vi "RQST Comm_Close All Connections.vi"(7 "Name":string, 8 "error in":errorcluster, 10 "ref in":T1, 11 "listener ID":refnum<k5>) -> (0 "error out":errorcluster)   [LabVIEW 2015, in "Diagnostics Addon Engine.lvlib"]
uses:
  Diagnostics Addon Engine.lvlib
  STM Lookup Table Ref.ctl
  Connection Manager/stm_TCPConnectionMethod.ctl
  <vilib>/NI Veristand/Custom Device Tools/Custom Device Utility Library/Custom Device Utility Library.lvlib
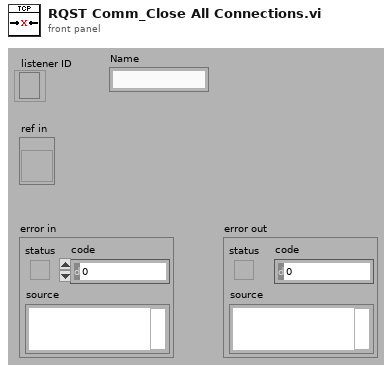
[diagram p1: front panel]
types:
  T1 = typedef "Diagnostics Addon Engine.lvlib/STM Lookup Table Ref.ctl" = refnum<vi>
  T2 = typedef "Diagnostics Addon Engine.lvlib/stm_TCPConnectionMethod.ctl" = enum16{"Initialize", "Add Connection", "Set Properties", "Get Connection(s)", "Remove Connection", "Remove All Connections", "Get Connection Count"}
  T3 = typedef "Diagnostics Addon Engine.lvlib/stm_TCP Connection Info.ctl" = cluster{"connection ID":refnum<k5>, "Meta data":T4[]}
  T4 = typedef "Diagnostics Addon Engine.lvlib/stm_MetaDataElement.ctl" = string
  T5 = typedef "Diagnostics Addon Engine.lvlib/stm_TCPConnectionProperties.ctl" = cluster{"Name":string, "Address":string, "Custom":string}
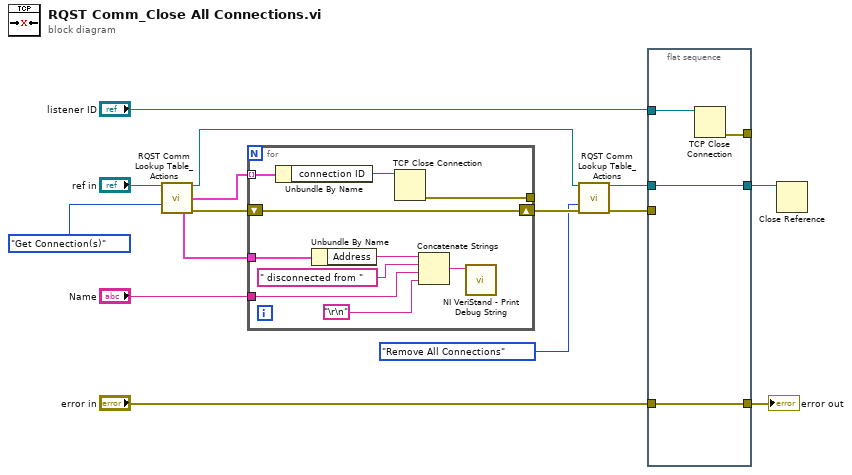
[diagram p0: block diagram]
diagram:
  n1 = call "RQST Comm Lookup Table_Actions.vi"("ref in"="ref in", "Method"=stm_TCPConnectionMethod."Get Connection(s)") -> ("ref out"=w3:T1, "All Connections"=w11:T3[], "Properties Out"=w1:T5, "error out"=w10:errorcluster)  [unwired: 7 in, 3 out]
  n2 = for {
    tunnel: w11 -> [w17] mode=indexing
    shift-right: [w23] -> w9
    shift-left: w10 -> [w23]
    tunnel: [w24] -> _
    tunnel: "Name" -> [w19]
    tunnel: w1 -> [w18]
    n3 = Unbundle By Name(w17) -> ("connection ID"=w25:refnum<k5>)
    n4 = Unbundle By Name(w18) -> ("Address"=w20:string)
    n5 = TCP Close Connection(connection ID=w25) -> (error out=w24:errorcluster)  [unwired: 2 in, 1 out]
    n6 = Concatenate Strings(w20, " disconnected from " ("string"), w19, "\r\n") -> (w22:string)
    n7 = call <vilib>:"NI VeriStand - Print Debug String.vi"("Message"=w22) -> ()  [unwired: 10 in, 1 out]
  }
  n8 = call "RQST Comm Lookup Table_Actions.vi"("ref in"=w3, "Method"=stm_TCPConnectionMethod."Remove All Connections", "error in (no error)"=w9) -> ("ref out"=w5:T1, "error out"=w8:errorcluster)  [unwired: 6 in, 5 out]
  n9 = flat-sequence {
    tunnel: "listener ID" -> [w29]
    tunnel: [w28] -> w14
    tunnel: w8 -> [_]
    tunnel: "error in" -> [w28]
    tunnel: [w27] -> _
    tunnel: w5 -> [w26]
    tunnel: [w26] -> w4
    frame #0 {
      n10 = TCP Close Connection(connection ID=w29) -> (error out=w27:errorcluster)  [unwired: 2 in, 1 out]
    }
  }
  n11 = Close Reference(reference=w4) -> ()  [unwired: 1 in, 1 out]
  "error out" <- w14
